vi "Load Test Case from File.vi"(8 "error in":errorcluster, 9 "Test Class Path":path) -> (0 "error out":errorcluster, 1 "Test":refnum<class>)   [LabVIEW 2011, in "VITesterUtilities.lvlib"]
uses:
  Libraries/VITesterUtilities.lvlib
panel:
  # "Copyright © 2007 James Kring, Inc. All rights reserved.\n\nAuthor: Omar Mussa [omar.mussa@jameskring.com]\n\nThis library is provided \"AS IS\" ,WITHOUT WARRANTIES OR \nCONDITIONS OF ANY KIND, either express or implied.\n\nJames Kring, Inc. -- http://www.jameskring.com"
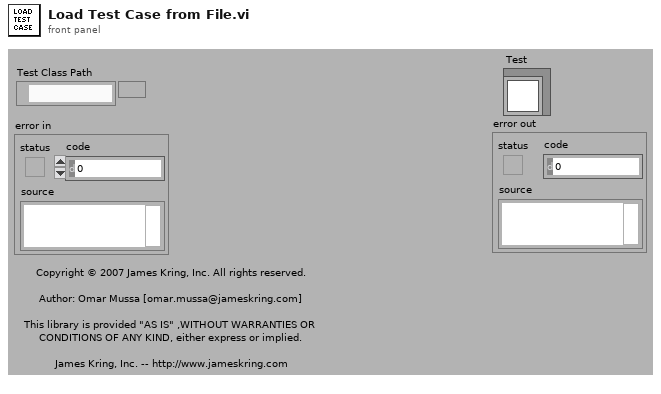
[diagram p1: front panel]
types:
  T1 = enum32{"invalid app kind", "Development System", "Run Time System", "Student Edition", "Embedded LabVIEW", "Evaluation", "Custom"}
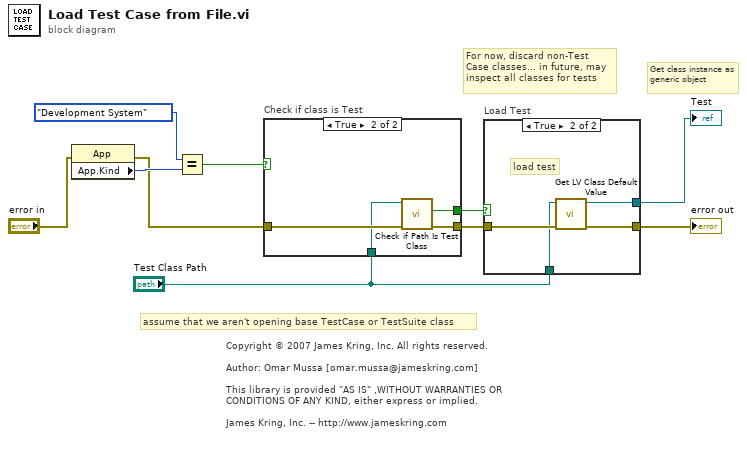
[diagram p0: block diagram]
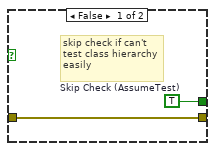
[diagram p2: hidden frame]
diagram:
  # "assume that we aren't opening base TestCase or TestSuite class"
  # "Get class instance as generic object"
  # "Copyright © 2007 James Kring, Inc. All rights reserved.\n\nAuthor: Omar Mussa [omar.mussa@jameskring.com]\n\nThis library is provided \"AS IS\" ,WITHOUT WARRANTIES OR \nCONDITIONS OF ANY KIND, either express or implied.\n\nJames Kring, Inc. -- http://www.jameskring.com"
  # "For now, discard non-Test Case classes... in future, may inspect all classes for tests"
  n1 = property class="App"(error in="error in") -> (error out=w1:errorcluster, "App.Kind"=w5:T1)  [unwired: 1 in, 1 out]
  n2 = Equal?(x=T1."Development System" ("y"), y=w5) -> (x = y?=w4:bool)
  n3 = case "Check if class is Test" shown="True" w4 {
    tunnel: w1 -> [w11 w16]
    tunnel: [w11 w15] -> w10
    tunnel: "Test Class Path" -> [_ w14]
    tunnel: [w12 w13] -> w7
    frame False {
      w12 = TRUE  # Skip Check (AssumeTest)
      # "skip check if can't\ntest class hierarchy\neasily"
    }
    frame True {
      n4 = call "Check if Path Is Test Class.vi"("error in"=w16, "Test Class Path"=w14) -> ("error out"=w15:errorcluster, "IsTestObject"=w13:bool)  [unwired: 7 in, 1 out]
    }
  }
  n5 = case "Load Test" shown="True" w7 {
    tunnel: w10 -> [w17 w21]
    tunnel: [w17 w20] -> w9
    tunnel: "Test Class Path" -> [_ w19]
    tunnel: [_ w18] -> w6
    frame False {
      # "do not load non\ntest objects"
    }
    frame True {
      # "load test"
      n6 = call <vilib>:"Get LV Class Default Value.vi"("error in (no error)"=w21, "class path"=w19) -> ("error out"=w20:errorcluster, "object"=w18:refnum<class>)  [unwired: 8 in]
    }
  }
  "error out" <- w9
  "Test" <- w6
